vi "創造圖片(2D).vi"(8 "error In":errorcluster, 10 "影像數量":i32=1, 11 "ImageNameArray":string[](array[string])=["Source"]) -> (0 "error out":errorcluster, 1 "ImageOutNameArray":string[](array[string]), 2 "ImageNameNumber":i32, 3 "Image2DArray":T1[][](array[typedef]))   [LabVIEW 2015]
uses:
  <vilib>/vision/Image Controls.llb/IMAQ Image.ctl
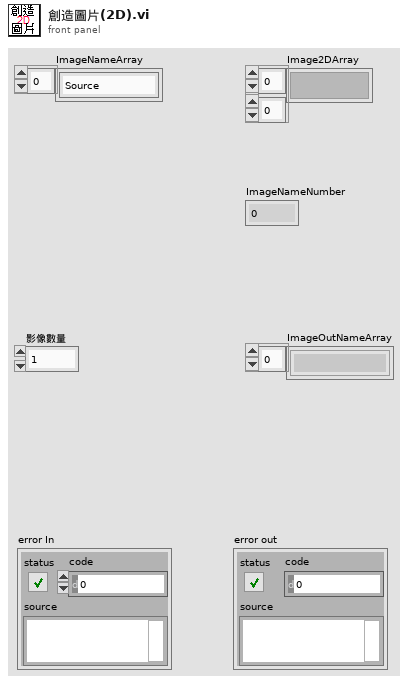
[diagram p1: front panel]
types:
  T1 = typedef "IMAQ Image.ctl" = refnum<image>
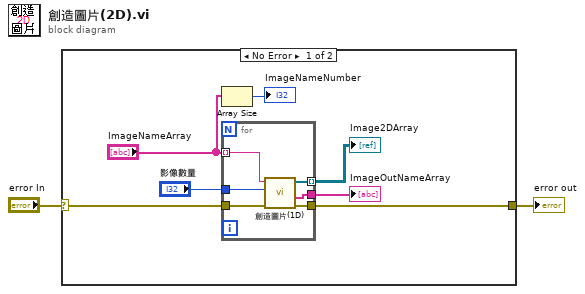
[diagram p0: block diagram]
diagram:
  n1 = case shown="No Error" "error In" {
    selector: "error In" -> [w3 w16]
    tunnel: [w8 w16] -> w2
    frame No Error {
      n2 = Array Size(array="ImageNameArray") -> (size(s)=→"ImageNameNumber":i32)
      n3 = for {
        tunnel: "ImageNameArray" -> [w15] mode=indexing
        tunnel: [w11] -> w9 mode=indexing
        tunnel: w3 -> [w13]
        tunnel: [w12] -> w8
        tunnel: "影像數量" -> [w14]
        tunnel: [w10] -> w4
        n4 = call "創造圖片(1D).vi"("error In"=w13, "影像數量"=w14, "Image Name"=w15) -> ("error out"=w12:errorcluster, "ImageOutNameArray"=w10:string[], "Image1DArray"=w11:T1[])  [unwired: 6 in]
      }
      "Image2DArray" <- w9
      "ImageOutNameArray" <- w4
    }
    frame Error {
    }
  }
  "error out" <- w2
